vi "Send Scope Report Event.vi"(7 "Message Priority (Normal)":T2=enum."Normal", 8 "error in (no error)":errorcluster, 9 "Event Data":variant, 10 "Scope Events":T1, 11 "Message Enqueuer":refnum<class "Message Enqueuer.lvclass">) -> (0 "error out":errorcluster, 3 "Message Enqueuer out":refnum<class "Message Enqueuer.lvclass">)   [LabVIEW 2020, in "Actor_Scope.lvlib" / "Scope Report Event Msg.lvclass"]
doc: "This VI sends the message to an actor."
uses:
  Scope Report Event Msg.lvclass
  <vilib>/ActorFramework/Message Enqueuer/Message Enqueuer.lvclass
  <vilib>/ActorFramework/Message Enqueuer/Message Priority.ctl
  Actor_Scope/Scope_Event.ctl
  C:/Program Files/National Instruments/LabVIEW 2020/vi.lib/ActorFramework/Message/Message.lvclass
  Scope Report Event Msg.lvclass/Scope Report Event Msg.ctl
  <vilib>/ActorFramework/Message Enqueuer/Message Enqueuer.lvclass/Message Enqueuer.ctl
  <vilib>/ActorFramework/Message Priority Queue/Priority Enqueue.vi
  Actor_Scope/Actor_Scope.lvclass
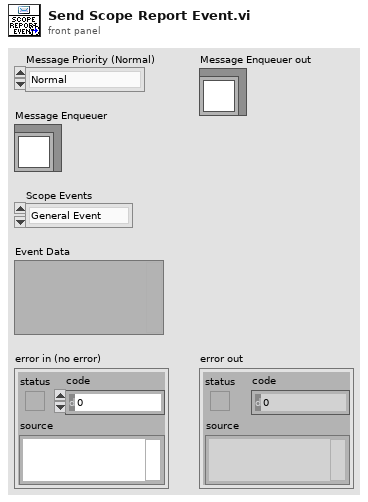
[diagram p1: front panel]
types:
  T1 = typedef "Actor_Scope.lvlib/Actor_Scope.lvclass/Scope_Event.ctl" = enum16{"General Event", "Inited", "Error", "Wfm Acq Complete"}
  T2 = typedef "Actor Framework.lvlib/Message Enqueuer.lvclass/Message Priority.ctl" = enum16{"Low", "Normal", "High"}
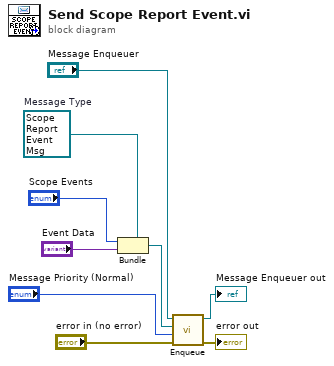
[diagram p0: block diagram]
diagram:
  w6 = refnum<class "Scope Report Event Msg.lvclass"> refnum  # Message Type
  n1 = Bundle(cluster=w6, "Scope Events", "Event Data") -> (w5:refnum<class "Scope Report Event Msg.lvclass">)
  n2 = call <vilib>:"Enqueue.vi"("error in (no error)"="error in (no error)", "Message Priority (Normal)"="Message Priority (Normal)", "Message"=w5, "Message Enqueuer in"="Message Enqueuer") -> ("error out"=→"error out":errorcluster, "Message Enqueuer out"=→"Message Enqueuer out":refnum<class "Message Enqueuer.lvclass">)  [unwired: 6 in]
